vi "CreateTask.vi"(0 "FPGA Ref in":refnum<k20>, 7 "session in":refnum<class "niInstr FIFO Register Bus v1 Host.lvclass">, 11 "error in":errorcluster) -> (4 "FPGA Ref out":refnum<k20>, 6 "Task out":refnum<class "WaveformTask.lvclass">, 8 "session out":refnum<class "niInstr FIFO Register Bus v1 Host.lvclass">, 15 "error out":errorcluster)   [LabVIEW 2015, in "WaveformTask.lvclass"]
uses:
  WaveformTask.lvclass
  <instrlib>/_niInstr/FIFO Register Bus/v1/Host/niInstr FIFO Register Bus v1 Host.lvclass
  DataFIFOs.ctl
  WaveformTask.lvclass/WaveformTask.ctl
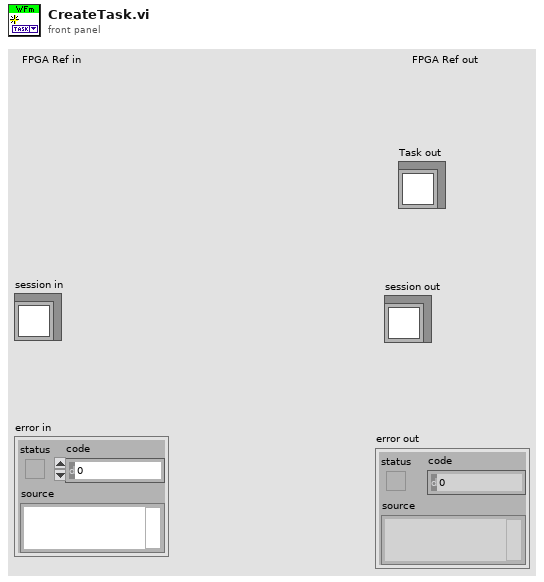
[diagram p1: front panel]
types:
  T1 = typedef "WaveformTask.lvclass/DataFIFOs.ctl" = refnum<k20>
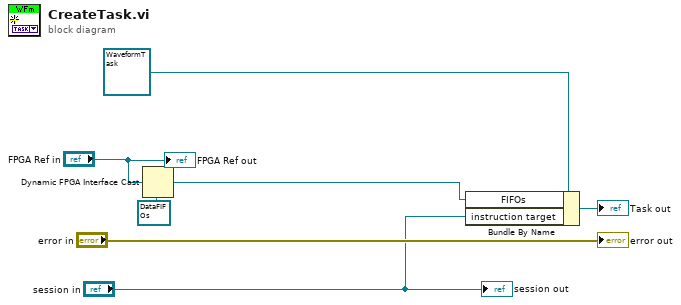
[diagram p0: block diagram]
diagram:
  n1 = Dynamic FPGA Interface Cast(Session In=T1 refnum ("FIFOs"), Type="FPGA Ref in") -> (Session Out=w4:T1)
  n2 = Bundle By Name(cluster=refnum<class "WaveformTask.lvclass"> refnum ("WaveformTask.lvclass"), "FIFOs"=w4, "instruction target"="session in") -> (→"Task out":refnum<class "WaveformTask.lvclass">)
  "FPGA Ref out" <- "FPGA Ref in"
  "error out" <- "error in"
  "session out" <- "session in"
